vi "WaveformFile, Create One-Pulse Burst.vi"(6 "error in":errorcluster, 9 "filename":path=path "C:/5-01-003 Active Electrode Min Max/One-Pulse Burst.dat") -> (0 "error out":errorcluster)   [LabVIEW 2010]
uses:
  Pulse Parameters.ctl
  <vilib>/Waveform/WDTFileIO.llb/ Write Waveform to File.vi
panel:
  in  "noise":dbl[unit]=0.02 min=0.0 step=0.1 format="%.3f"
  in  "burst count":i32=8 min=1 step=1
  in  "frequency":dbl[unit]=234.0 format="%.1f"
  in  "save file (T)":bool=TRUE
  in  "waveform in":waveform(dbl)={"t0"=timestamp(3474892848.0780005 s since 1904-01-01), "dt"=1e-07, "Y"=[]}
  out "waveform":waveform(dbl)(graph)={"t0"=timestamp(3474892848.0780005 s since 1904-01-01), "dt"=1e-07, "Y"=[]}
  in  "Recovery Phase":T1={"offset"=0.0, "amplitude"=-2.0, "delay"=4.9999999999999996e-05, "leading edge"=2.4999999999999998e-05, "pulse width"=0.0003, "trailing edge"=2.4999999999999998e-05, "ref level %"=33.333} {"ref level %" format="%.3f"; "offset" format="%.3f"; "pulse width" format="%.1f"; "trailing edge" format="%.1f"; "amplitude" format="%.3f"; "delay" format="%.1f"; "leading edge" format="%.1f"}
  in  "Stimulus Phase":T1={"offset"=0.0, "amplitude"=2.001, "delay"=0.00019999999999999998, "leading edge"=4.9999999999999996e-05, "pulse width"=0.00039999999999999996, "trailing edge"=4.9999999999999996e-05, "ref level %"=33.333} {"ref level %" format="%.3f"; "offset" format="%.3f"; "pulse width" format="%.1f"; "trailing edge" format="%.1f"; "amplitude" format="%.3f"; "delay" format="%.1f"; "leading edge" format="%.1f"}
  in  "append file (F)":bool
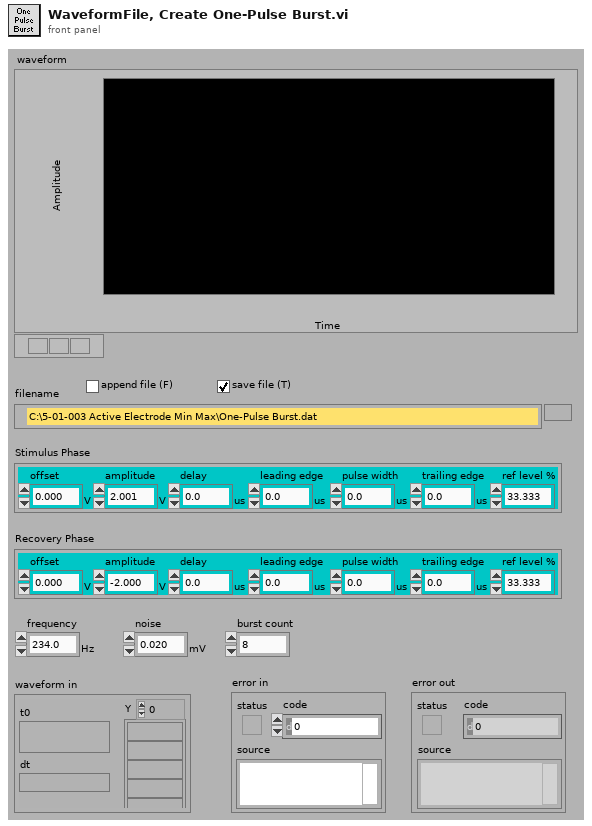
[diagram p1: front panel]
types:
  T1 = typedef "Pulse Parameters.ctl" = cluster{"offset":dbl[unit], "amplitude":dbl[unit], "delay":dbl[unit], "leading edge":dbl[unit], "pulse width":dbl[unit], "trailing edge":dbl[unit], "ref level %":dbl}
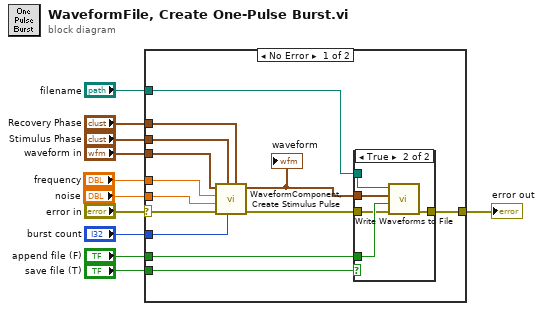
[diagram p0: block diagram]
diagram:
  n1 = case shown="No Error" "error in" {
    selector: "error in" -> [w16 w31]
    tunnel: "waveform in" -> [w20 _]
    tunnel: "Stimulus Phase" -> [w19 _]
    tunnel: "Recovery Phase" -> [w18 _]
    tunnel: [w24 w31] -> w8
    tunnel: "filename" -> [w23 _]
    tunnel: "append file (F)" -> [w22 _]
    tunnel: "save file (T)" -> [w21 _]
    tunnel: "frequency" -> [w17 _]
    tunnel: "burst count" -> [w13 _]
    tunnel: "noise" -> [w12 _]
    frame No Error {
      n2 = call "WaveformComponent, Create Stimulus Pulse.vi"("Recovery Phase"=w18, "burst count (1)"=w13, "Stimulus Phase"=w19, "error in"=w16, "noise (0.1)"=w12, "frequency"=w17, "waveform in"=w20) -> ("error out"=w15:errorcluster, "waveform out"=w14:waveform(dbl))  [unwired: 3 in]
      "waveform" <- w14
      n3 = case shown="True" w21 {
        tunnel: [w25 w30] -> w24
        tunnel: w23 -> [_ w29]
        tunnel: w22 -> [_ w28]
        tunnel: w15 -> [w25 w27]
        tunnel: w14 -> [_ w26]
        frame False {
        }
        frame True {
          n4 = call-poly <vilib>:"Write Waveforms to File.vi"("error in (no error)"=w27, "append to file? (new file:F)"=w28, "waveform"=w26, "file path (dialog if empty)"=w29) -> ("error out"=w30:errorcluster)  [unwired: 6 in, 1 out]
        }
      }
    }
    frame Error {
    }
  }
  "error out" <- w8
